vi "Write Element of TRH.vi"(8 "error in":errorcluster, 9 "TRH [i]":sgl, 10 "index":i32, 11 "CRDS Data in":refnum<class "CRDS Data.lvclass">) -> (0 "error out":errorcluster, 3 "CRDS Data out":refnum<class "CRDS Data.lvclass">)   [LabVIEW 2011, in "CRDS Data.lvclass"]
uses:
  CRDS Data.lvclass
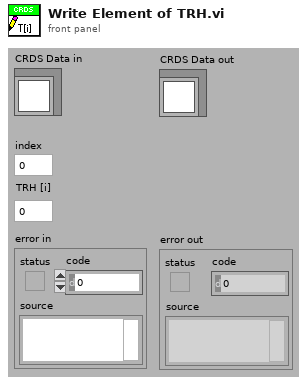
[diagram p1: front panel]
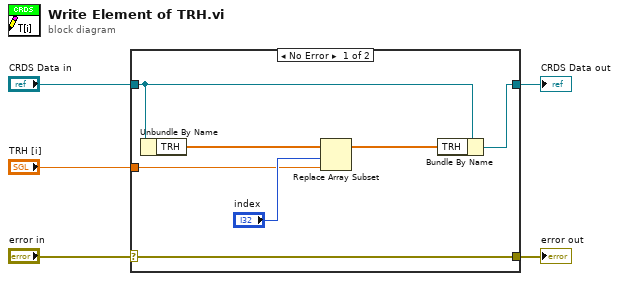
[diagram p0: block diagram]
diagram:
  n1 = case shown="No Error" "error in" {
    selector: "error in" -> [w12 w13]
    tunnel: [w12 w13] -> w4
    tunnel: [w11 w14] -> w2
    tunnel: "CRDS Data in" -> [w10 w14]
    tunnel: "TRH [i]" -> [w6 _]
    frame No Error {
      n2 = Unbundle By Name(w10) -> ("TRH"=w9:sgl[])
      n3 = Replace Array Subset(array=w9, new element=w6, index="index") -> (w8:sgl[])
      n4 = Bundle By Name(cluster=w10, "TRH"=w8) -> (w11:refnum<class "CRDS Data.lvclass">)
    }
    frame Error {
    }
  }
  "error out" <- w4
  "CRDS Data out" <- w2
